vi "SetProgressValue.vi"(7 "maximum (100)":u64=100, 8 "error in (no error)":errorcluster, 10 "current (0)":u64, 11 "Window Handle":refnum<k24>) -> (0 "error out":errorcluster, 3 "dup Window Handle":refnum<k24>)   [LabVIEW 2020, in "Progress Bar.lvclass"]
uses:
  <userlib>/_MGI/User Interface/Progress Bar/Progress Bar.lvclass
  C:/Program Files/National Instruments/LabVIEW 2020/user.lib/_MGI/User Interface/Progress Bar/Windows7 Taskbar API/Windows7Taskbar_LV9.dll
  Windows7Taskbar_LV9.dll
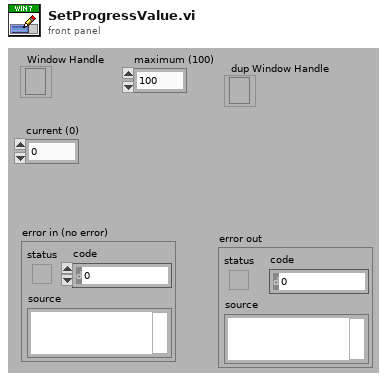
[diagram p1: front panel]
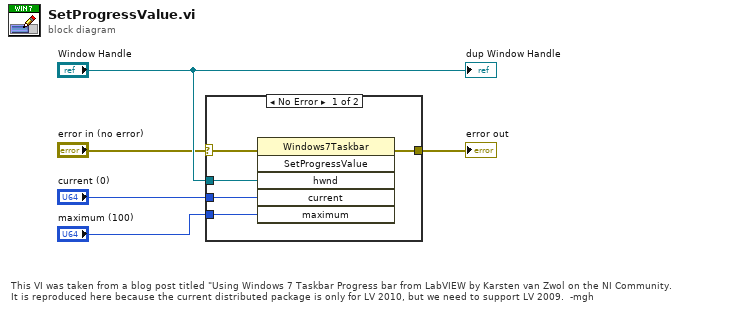
[diagram p0: block diagram]
diagram:
  # "This VI was taken from a blog post titled \"Using Windows 7 Taskbar Progress bar from LabVIEW by Karsten van Zwol on the NI Community.\nIt is reproduced here because the current distributed package is only for LV 2010, but we need to support LV 2009.  -mgh"
  n1 = case shown="No Error" "error in (no error)" {
    selector: "error in (no error)" -> [w8 w11]
    tunnel: [w10 w11] -> w5
    tunnel: "Window Handle" -> [w9 _]
    tunnel: "current (0)" -> [w7 _]
    tunnel: "maximum (100)" -> [w6 _]
    frame No Error {
      n2 = invoke class="Windows7Taskbar" method="SetProgressValue"(error in=w8, "hwnd"=w9, "current"=w7, "maximum"=w6) -> (error out=w10:errorcluster)  [unwired: 2 in, 5 out]
    }
    frame Error {
    }
  }
  "error out" <- w5
  "dup Window Handle" <- "Window Handle"
